vi "Get Number of Objects.vi"(4 "# Objects":i32) -> (1 "# Objects":i32)   [LabVIEW 2020, in "CBOR.lvlib"]
doc: "Convert All(-1) into I32 max value(2147483647)."
uses:
  CBOR.lvlib
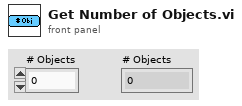
[diagram p1: front panel]
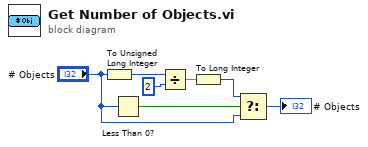
[diagram p0: block diagram]
diagram:
  n1 = To Unsigned Long Integer(number="# Objects") -> (unsigned 32bit integer=w7:u32)
  n2 = Less Than 0?(x="# Objects") -> (x < 0?=w4:bool)
  n3 = Divide(x=w7, y=u32 2) -> (x/y=w5:dbl)
  n4 = To Long Integer(number=w5) -> (32bit integer=w3:i32)
  n5 = Select(t=w3, s=w4, f="# Objects") -> (s? t:f=→"# Objects":i32)
